vi "Get QMH Payload.vi"(8 "error in":errorcluster, 11 "IMessagePayload in":refnum<class "IMessagePayload.lvclass">) -> (0 "error out":errorcluster, 2 "QMH Payload":cluster{"State":enum16{""}, "Data":variant}, 3 "IMessagePayload":refnum<class "IMessagePayload.lvclass">)   [LabVIEW 2016, in "QMHMessagePayload.lvclass"]
uses:
  QMHMessagePayload.lvclass
  IMessagePayload/IMessagePayload.lvclass
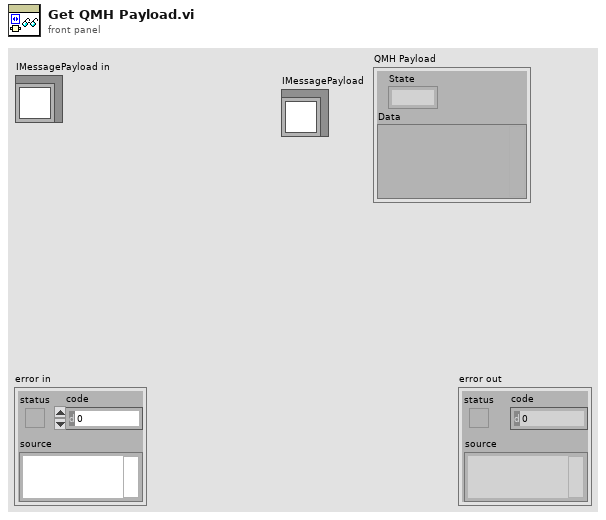
[diagram p1: front panel]
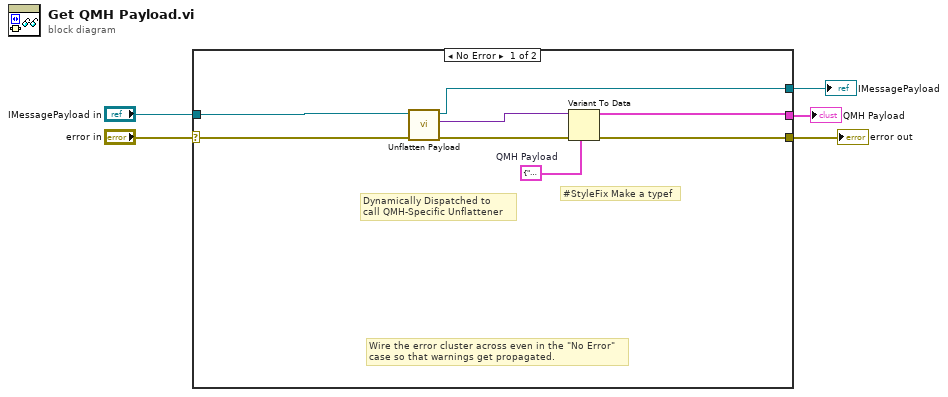
[diagram p0: block diagram]
diagram:
  n1 = case shown="No Error" "error in" {
    selector: "error in" -> [w12 w14]
    tunnel: [w8 w14] -> w4
    tunnel: "IMessagePayload in" -> [w13 _]
    tunnel: [w7 _] -> w2
    tunnel: [w6 _] -> w1
    frame No Error {
      w11 = cluster{"State":enum16{""}, "Data":variant} {"State"=enum."", "Data"=variant}  # QMH Payload
      # "#StyleFix Make a typef"
      # "Dynamically Dispatched to \ncall QMH-Specific Unflattener"
      # "Wire the error cluster across even in the \"No Error\"\ncase so that warnings get propagated."
      n2 = call-dynamic "Unflatten Payload.vi"("error in (no error)"=w12, "IMessagePayload in"=w13) -> ("error out"=w9:errorcluster, "Payload"=w10:variant, "IMessagePayload out"=w7:refnum<class "IMessagePayload.lvclass">)  [unwired: 7 in]
      n3 = Variant To Data(error in=w9, type=w11, Variant=w10) -> (data=w6:cluster{"State":enum16{""}, "Data":variant}, error out=w8:errorcluster)
    }
    frame Error {
    }
  }
  "error out" <- w4
  "IMessagePayload" <- w2
  "QMH Payload" <- w1
